vi "_unittest Assert Equal.vi"(4 "Ignore Error? (F)":bool, 6 "Assert Error Code (0=No error)":i32, 7 "Test Name":string, 8 "error in (no error)":errorcluster, 10 "Expected Value":variant, 11 "Actual Value":variant) -> (0 "error out":errorcluster, 2 "Passed?":bool, 3 "Summary":string)   [LabVIEW 2018, in "labview_json_tests.lvlib"]
uses:
  labview_json_tests.lvlib
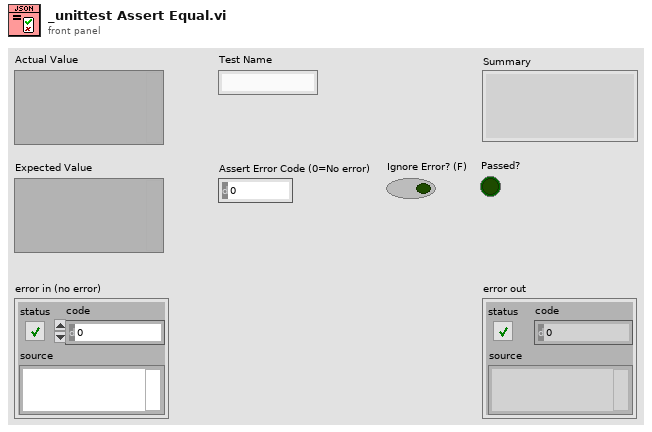
[diagram p1: front panel]
types:
  T1 = enum8{"Report", "Add Test Group", "Add Test Case"}
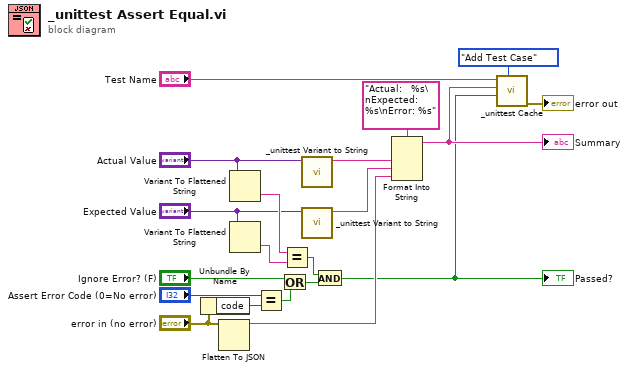
[diagram p0: block diagram]
diagram:
  n1 = Unbundle By Name("error in (no error)") -> ("code"=w20:i32)
  n2 = Flatten To JSON(anything="error in (no error)") -> (JSON string=w9:string)  [unwired: 2 in, 1 out]
  n3 = Variant To Flattened String(Variant="Actual Value") -> (data string=w6:string)  [unwired: 1 out]
  n4 = Variant To Flattened String(Variant="Expected Value") -> (data string=w5:string)  [unwired: 1 out]
  n5 = Equal?(x="Assert Error Code (0=No error)", y=w20) -> (x = y?=w14:bool)
  n6 = Or(x="Ignore Error? (F)", y=w14) -> (x .or. y?=w17:bool)
  n7 = Equal?(x=w6, y=w5) -> (x = y?=w16:bool)
  n8 = call "_unittest Variant to String.vi"("Actual Value"="Actual Value") -> ("String"=w11:string)  [unwired: 8 in, 2 out]
  n9 = call "_unittest Variant to String.vi"("Actual Value"="Expected Value") -> ("String"=w10:string)  [unwired: 8 in, 2 out]
  n10 = And(x=w16, y=w17) -> (x .and. y?=w3:bool)
  "Passed?" <- w3
  n11 = Format Into String(format string="Actual:   %s\nExpected: %s\nError: %s", w11, w10, w9) -> (resulting string=w7:string)  [unwired: 2 in, 1 out]
  "Summary" <- w7
  n12 = call "_unittest Cache.vi"("Action"=T1."Add Test Case", "Passed?"=w3, "Test Details"=w7, "Test Name"="Test Name") -> ("error out"=→"error out":errorcluster)  [unwired: 6 in, 1 out]
